vi "GetPropertyInfo.vi"(7 "property":string, 8 "enums":T6[](array[typedef]), 9 "scales":T4[](array[typedef]), 10 "registers":T2[](array[typedef]), 11 "properties":T1[](array[typedef])) -> (3 "property info":T8)   [LabVIEW 2017]
uses:
  Ctrl/ScaleType.ctl
  Ctrl/Scale.ctl
  Ctrl/EnumValue.ctl
  Ctrl/Enum.ctl
  Ctrl/Bitfield.ctl
  Ctrl/Register.ctl
  Ctrl/Property.ctl
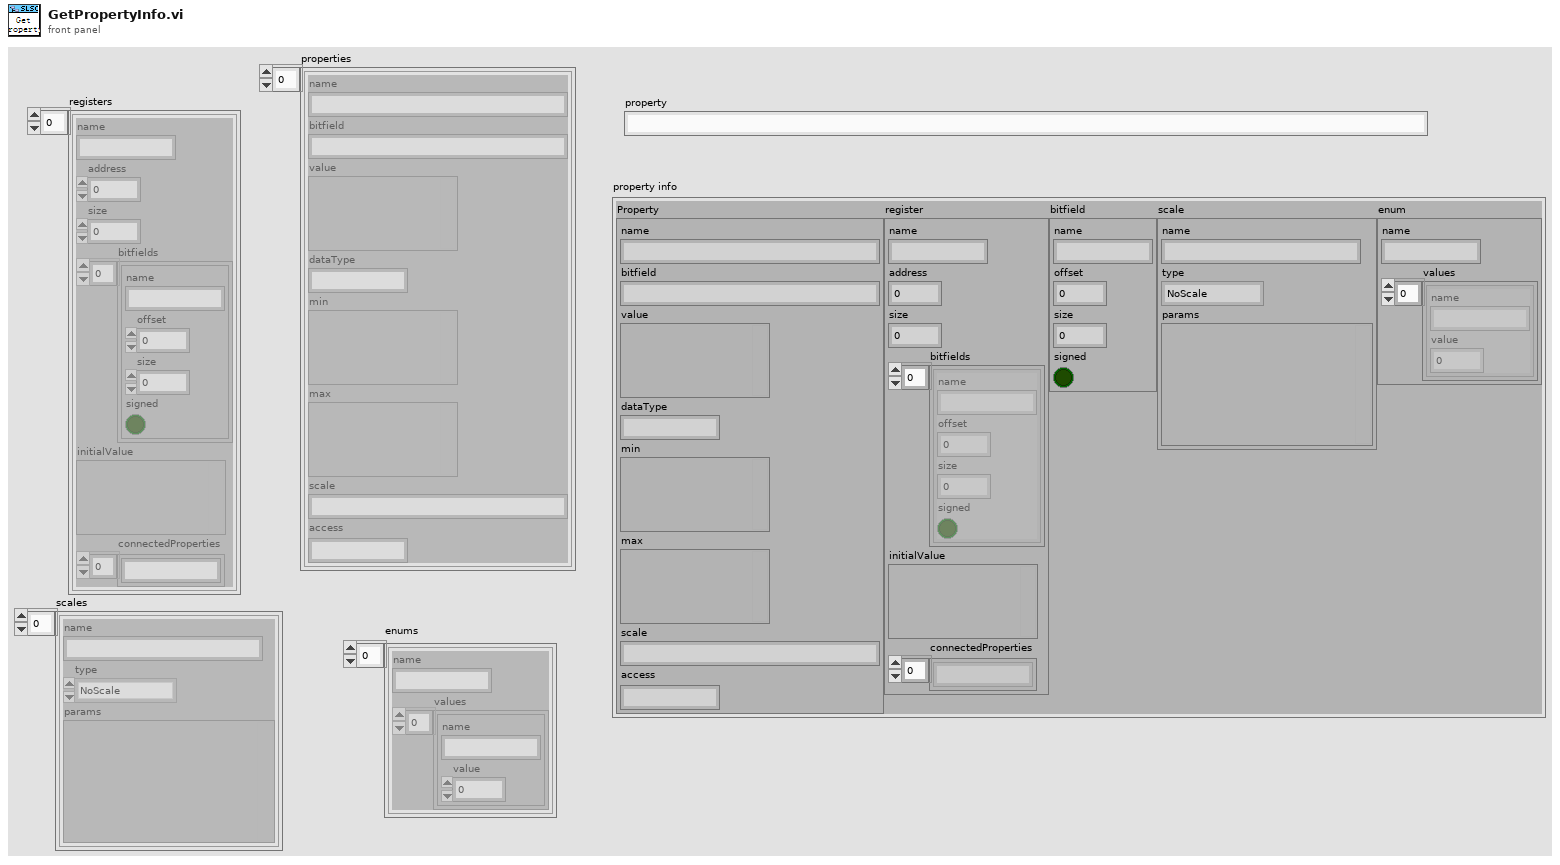
[diagram p1: front panel]
types:
  T1 = typedef "Property.ctl" = cluster{"name":string, "bitfield":string, "value":variant, "dataType":string, "min":variant, "max":variant, "scale":string, "access":string}
  T2 = typedef "Register.ctl" = cluster{"name":string, "address":i32, "size":i32, "bitfields":T3[], "initialValue":variant, "connectedProperties":string[]}
  T3 = typedef "Bitfield.ctl" = cluster{"name":string, "offset":i32, "size":i32, "signed":bool}
  T4 = typedef "Scale.ctl" = cluster{"name":string, "type":T5, "params":variant}
  T5 = typedef "ScaleType.ctl" = enum16{"NoScale", "Table", "Polynomial", "Linear"}
  T6 = typedef "Enum.ctl" = cluster{"name":string, "values":T7[]}
  T7 = typedef "EnumValue.ctl" = cluster{"name":string, "value":i32}
  T8 = cluster{"Property":T1, "register":T2, "bitfield":T3, "scale":T4, "enum":T6}
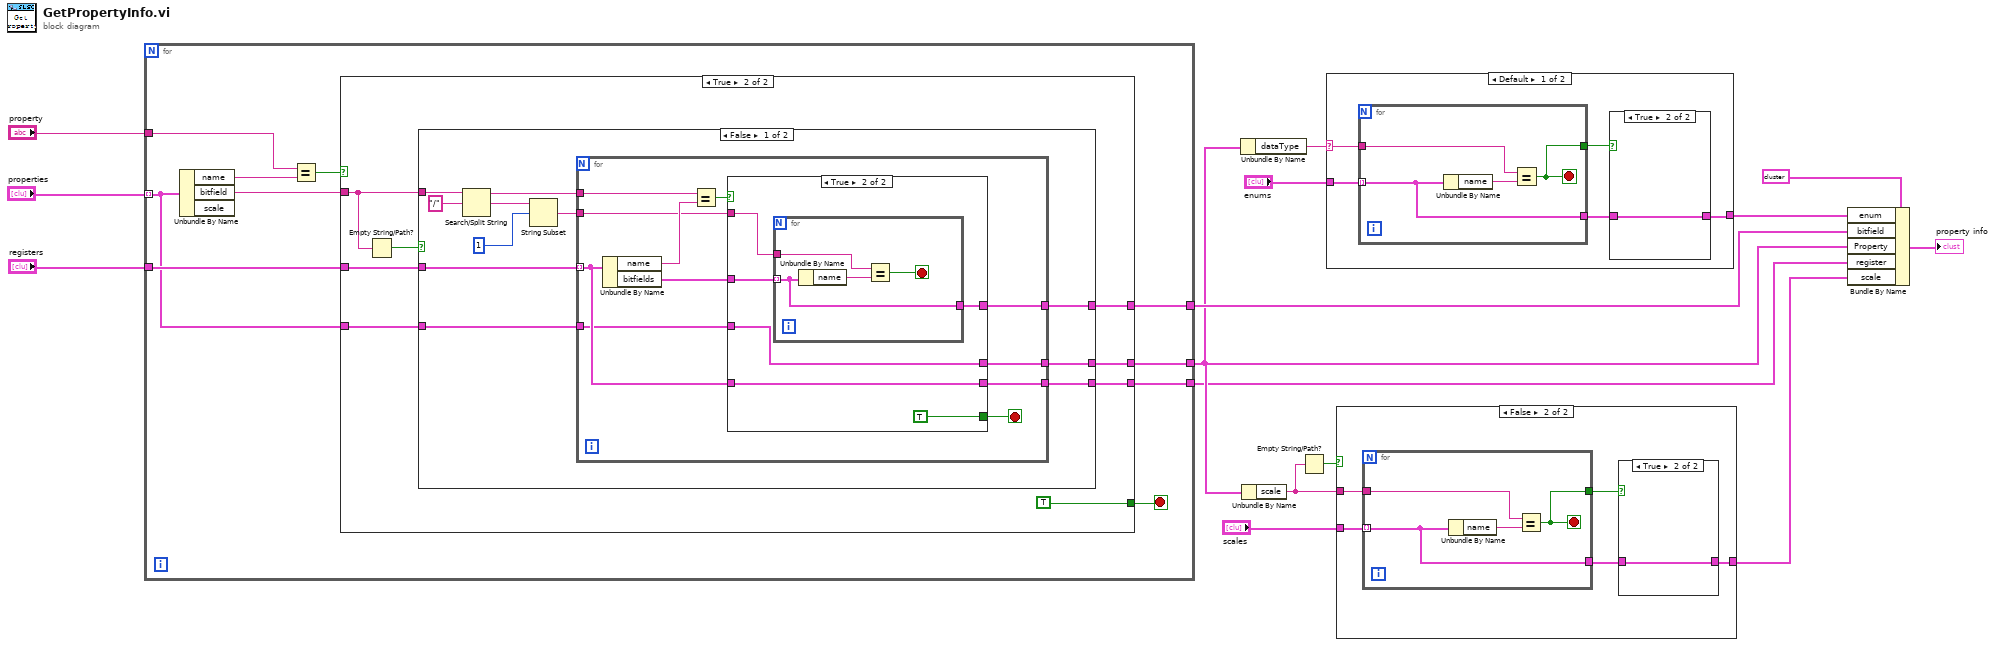
[diagram p0: block diagram]
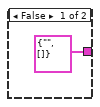
[diagram p2: hidden frame]
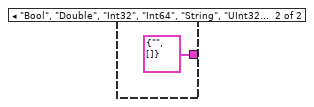
[diagram p3: hidden frame]
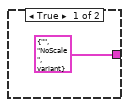
[diagram p4: hidden frame]
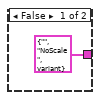
[diagram p5: hidden frame]
diagram:
  n1 = for {
    tunnel: "properties" -> [w19] mode=indexing
    tunnel: "property" -> [w24]
    tunnel: "registers" -> [w21]
    tunnel: [w18] -> w4
    tunnel: [w17] -> w5
    tunnel: [w16] -> w3
    stop <- w20 stop-if-true
    n2 = Unbundle By Name(w19) -> ("name"=w25:string, "bitfield"=w22:string)  [unwired: 1 out]
    n3 = Equal?(x=w24, y=w25) -> (x = y?=w23:bool)
    n4 = case shown="True" w23 {
      tunnel: w22 -> [_ w34]
      tunnel: w21 -> [_ w32]
      tunnel: [_ TRUE] -> w20
      tunnel: w19 -> [w26 w30]
      tunnel: [w26 w29] -> w18
      tunnel: [_ w28] -> w17
      tunnel: [_ w27] -> w16
      frame False {
      }
      frame True {
        n5 = Empty String/Path?(string/path=w34) -> (empty?=w33:bool)
        n6 = case shown="False" w33 {
          tunnel: w34 -> [w45 _]
          tunnel: w32 -> [w41 _]
          tunnel: w30 -> [w36 w67]
          tunnel: [w35 w67] -> w29
          tunnel: [w38 _] -> w28
          tunnel: [w37 _] -> w27
          frame False {
            n7 = Search/Split String(string=w45, search string/char (-)="/") -> (substring before match=w40:string, match + rest of string=w43:string)  [unwired: 1 in, 1 out]
            n8 = String Subset(string=w43, offset (0)=1) -> (substring=w39:string)  [unwired: 1 in]
            n9 = for {
              tunnel: w41 -> [w49] mode=indexing
              tunnel: w40 -> [w56]
              tunnel: w39 -> [w53]
              tunnel: [w50] -> w38
              tunnel: [w48] -> w37
              tunnel: w36 -> [w47]
              tunnel: [w46] -> w35
              stop <- w51 stop-if-true
              n10 = Unbundle By Name(w49) -> ("name"=w55:string, "bitfields"=w52:T3[])
              n11 = Equal?(x=w56, y=w55) -> (x = y?=w54:bool)
              n12 = case shown="True" w54 {
                tunnel: w53 -> [_ w61]
                tunnel: w52 -> [_ w62]
                tunnel: [_ TRUE] -> w51
                tunnel: [_ w59] -> w50
                tunnel: w49 -> [_ w58]
                tunnel: [_ w58] -> w48
                tunnel: w47 -> [_ w57]
                tunnel: [_ w57] -> w46
                frame False {
                }
                frame True {
                  n13 = for {
                    tunnel: w62 -> [w63] mode=indexing
                    tunnel: w61 -> [w65]
                    tunnel: [w63] -> w59
                    stop <- w64 stop-if-true
                    n14 = Unbundle By Name(w63) -> ("name"=w66:string)
                    n15 = Equal?(x=w65, y=w66) -> (x = y?=w64:bool)
                  }
                }
              }
            }
          }
          frame True {
          }
        }
      }
    }
  }
  n16 = Unbundle By Name(w4) -> ("dataType"=w9:string)
  n17 = Unbundle By Name(w4) -> ("scale"=w11:string)
  n18 = Empty String/Path?(string/path=w11) -> (empty?=w10:bool)
  n19 = case shown="Default" w9 {
    selector: w9 -> [w71 _]
    tunnel: "enums" -> [w72 _]
    tunnel: [w68 T6 {"name"="", "values"=[]} ("Enum")] -> w6
    frame Default {
      n20 = for {
        tunnel: w71 -> [w78]
        tunnel: w72 -> [w76] mode=indexing
        tunnel: [w76] -> w70
        tunnel: [w75] -> w69
        stop <- w75 stop-if-true
        n21 = Unbundle By Name(w76) -> ("name"=w77:string)
        n22 = Equal?(x=w78, y=w77) -> (x = y?=w75:bool)
      }
      n23 = case shown="True" w69 {
        tunnel: w70 -> [_ w74]
        tunnel: [T6 {"name"="", "values"=[]} ("Enum") w74] -> w68
        frame False {
        }
        frame True {
        }
      }
    }
    frame "Bool", "Double", "Int32", "Int64", "String", "UInt32", "UInt64" {
    }
  }
  n24 = case shown="False" w10 {
    tunnel: w11 -> [_ w85]
    tunnel: "scales" -> [_ w84]
    tunnel: [T4 {"name"="", "type"=enum."NoScale", "params"=variant} w81] -> w2
    frame True {
    }
    frame False {
      n25 = for {
        tunnel: w85 -> [w91]
        tunnel: w84 -> [w89] mode=indexing
        tunnel: [w89] -> w82
        tunnel: [w88] -> w83
        stop <- w88 stop-if-true
        n26 = Unbundle By Name(w89) -> ("name"=w90:string)
        n27 = Equal?(x=w91, y=w90) -> (x = y?=w88:bool)
      }
      n28 = case shown="True" w83 {
        tunnel: w82 -> [_ w87]
        tunnel: [T4 {"name"="", "type"=enum."NoScale", "params"=variant} w87] -> w81
        frame False {
        }
        frame True {
        }
      }
    }
  }
  n29 = Bundle By Name(cluster=T8 {"Property"={"name"="", "bitfield"="", "value"=variant, "dataType"="", "min"=variant, "max"=variant, "scale"="", "access"=""}, "register"={"name"="", "address"=0, "size"=0, "bitfields"=[], "initialValue"=variant, "connectedProperties"=[]}, "bitfield"={"name"="", "offset"=0, "size"=0, "signed"=FALSE}, "scale"={"name"="", "type"=enum."NoScale", "params"=variant}, "enum"={"name"="", "values"=[]}} ("property info"), "enum"=w6, "bitfield"=w5, "Property"=w4, "register"=w3, "scale"=w2) -> (→"property info":T8)
